vi "Position Open Mission Cancel Button.vi"(8 "error in (no error)":errorcluster, 11 "Button Ref":refnum<vi>) -> (0 "error out":errorcluster)   [LabVIEW 2014]
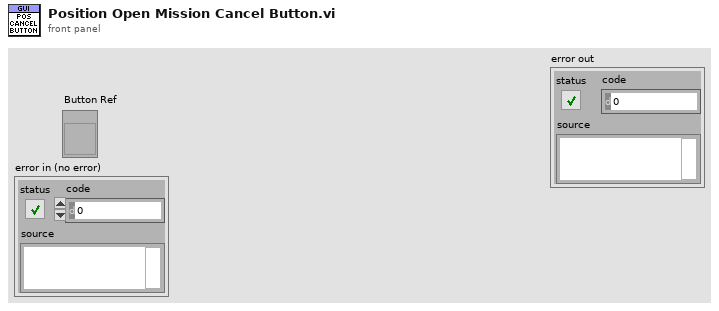
[diagram p1: front panel]
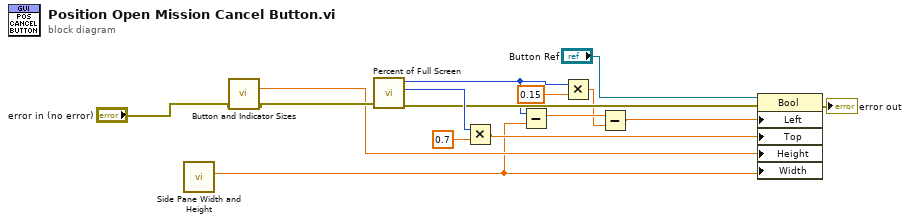
[diagram p0: block diagram]
diagram:
  n1 = call "Side Pane Width and Height.vi"() -> ("Width"=w7:dbl)  [unwired: 9 in, 2 out]
  n2 = call "Button and Indicator Sizes.vi"("error in (no error)"="error in (no error)") -> ("Button Height"=w11:dbl, "error out"=w13:errorcluster)  [unwired: 10 in, 3 out]
  n3 = call "Percent of Full Screen.vi"("error in (no error)"=w13) -> ("error out"=w6:errorcluster, "Bottom"=w8:i16, "Right"=w5:i16)  [unwired: 8 in]
  n4 = Multiply(x=w8, y=0.7) -> (x*y=w9:dbl)
  n5 = Subtract(x=w5, y=w7) -> (x-y=w3:dbl)
  n6 = Multiply(x=w5, y=0.15) -> (x*y=w2:dbl)
  n7 = Subtract(x=w3, y=w2) -> (x-y=w1:dbl)
  n8 = property class="Bool"(reference="Button Ref", error in=w6, "Left"=w1, "Top"=w9, "Height"=w11, "Width"=w7) -> (error out=→"error out":errorcluster)  [unwired: 1 out]
